vi "Suite.vi"(8 "error in (no error)":errorcluster, 10 "LUnit Test Suite in":refnum<class "LUnit Test Suite.lvclass">, 11 "LUnit Test Case In":refnum<class "LUnit Test Case.lvclass">) -> (0 "error out":errorcluster, 2 "LUnit Test Suite Out":refnum<class "LUnit Test Suite.lvclass">, 3 "LUnit Test Case Out":refnum<class "LUnit Test Case.lvclass">)   [LabVIEW 2020, in "LUnit Test Case.lvclass"]
doc: "Factory method to generate a Test Suite object for the test case class.\nThe Test Suite input is used as a collecting parameter to which the test case methods are appended. This can be useful when using custom test suite classes."
uses:
  LUnit Test Case.lvclass
  C:/git/astemes-lunit/source/Core/Runnable/Runnable.lvclass
  LUnit Test Suite.lvclass
  LUnit Test Case.lvclass/LUnit Test Case.ctl
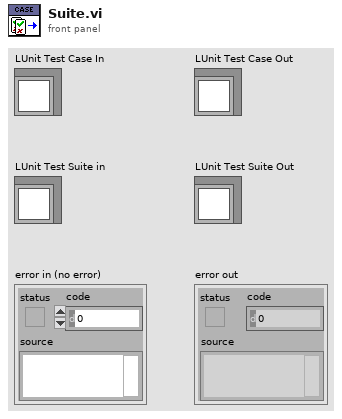
[diagram p1: front panel]
types:
  T1 = enum32{"invalid scope", "public", "private", "protected", "community"}
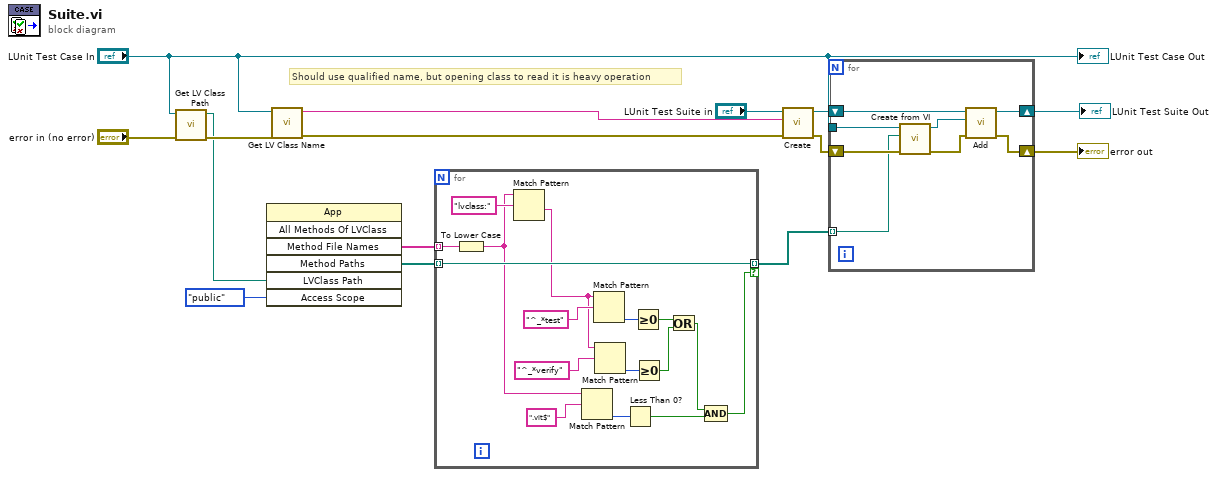
[diagram p0: block diagram]
diagram:
  # "Should use qualified name, but opening class to read it is heavy operation"
  n1 = call <vilib>:"Get LV Class Path.vi"("error in (no error)"="error in (no error)", "object"="LUnit Test Case In") -> ("error out"=w5:errorcluster, "class path"=w2:path)  [unwired: 8 in]
  n2 = invoke class="App" method="All Methods Of LVClass"("LVClass Path"=w2, "Access Scope"=T1."public") -> ("Method File Names"=w3:string[], "Method Paths"=w6:path[])  [unwired: 5 in, 5 out]
  n3 = call <vilib>:"Get LV Class Name.vi"("error in (no error)"=w5, "object"="LUnit Test Case In") -> ("error out"=w4:errorcluster, "class name"=w1:string)  [unwired: 8 in]
  n4 = for {
    tunnel: [w27] -> w15 mode=indexing if=w28
    tunnel: w6 -> [w27] mode=indexing
    tunnel: w3 -> [w23] mode=indexing
    n5 = To Lower Case(string=w23) -> (all lower case string=w16:string)
    n6 = Match Pattern(string=w16, regular expression="lvclass:") -> (after substring=w24:string)  [unwired: 1 in, 3 out]
    n7 = Match Pattern(string=w16, regular expression=".vit$") -> (offset past match=w30:i32)  [unwired: 1 in, 3 out]
    n8 = Match Pattern(string=w24, regular expression="^_*test") -> (offset past match=w26:i32)  [unwired: 1 in, 3 out]
    n9 = Match Pattern(string=w24, regular expression="^_*verify") -> (offset past match=w20:i32)  [unwired: 1 in, 3 out]
    n10 = Less Than 0?(x=w30) -> (x < 0?=w29:bool)
    n11 = Greater Or Equal To 0?(x=w26) -> (x >= 0?=w17:bool)
    n12 = Greater Or Equal To 0?(x=w20) -> (x >= 0?=w19:bool)
    n13 = Or(x=w17, y=w19) -> (x .or. y?=w18:bool)
    n14 = Compound Arithmetic op=AND(w18, w29) -> (w28:bool)
  }
  n15 = call "Create.vi"("error in (no error)"=w4, "Suite Name"=w1, "LUnit Test Suite in"="LUnit Test Suite in") -> ("error out"=w13:errorcluster, "LUnit Test Suite Out"=w14:refnum<class "LUnit Test Suite.lvclass">)  [unwired: 7 in]
  n16 = for {
    tunnel: w15 -> [w32] mode=indexing
    shift-right: [w38] -> w12
    shift-left: w14 -> [w39]
    shift-right: [w36] -> w10
    shift-left: w13 -> [w35]
    tunnel: "LUnit Test Case In" -> [w33]
    n17 = call "Create from VI.vi"("error in (no error)"=w35, "Test Method VI Path"=w32, "LUnit Test Case In"=w33) -> ("error out"=w37:errorcluster, "LUnit Test Case Out"=w34:refnum<class "LUnit Test Case.lvclass">)  [unwired: 7 in]
    n18 = call "Add.vi"("error in (no error)"=w37, "Runnable"=w34, "LUnit Test Suite In"=w39) -> ("error out"=w36:errorcluster, "LUnit Test Suite Out"=w38:refnum<class "LUnit Test Suite.lvclass">)  [unwired: 7 in]
  }
  "error out" <- w10
  "LUnit Test Suite Out" <- w12
  "LUnit Test Case Out" <- "LUnit Test Case In"
